vi "check_machine_limit.vi"(3 "input_machine_reference.lvclass":refnum<class "machine.lvclass">) -> (1 "output_machine_reference.lvclass":refnum<class "machine.lvclass">)   [LabVIEW 2014, in "machine.lvclass"]
uses:
  machine.lvclass
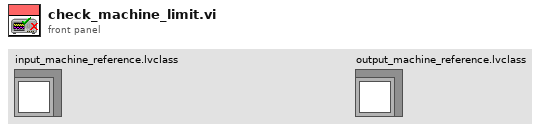
[diagram p1: front panel]
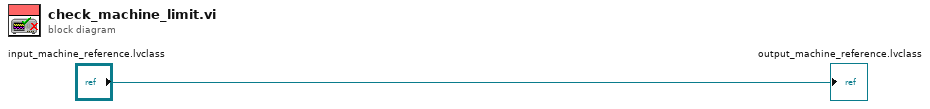
[diagram p0: block diagram]
diagram:
  "output_machine_reference.lvclass" <- "input_machine_reference.lvclass"
